vi "UI V7.1.2b.vi"() -> ()   [LabVIEW 2017]
uses:
  <vilib>/Instr/_visa.llb/VISA Configure Serial Port (Instr).vi
  <vilib>/addons/Biomedical/Biosignal Measurements/Biosignal Preprocessing/Biosignal Rate Extractor (Waveform).vi
  <vilib>/addons/Biomedical/NI_BMTK_Measurements.lvlib
panel:
  in  "?":refnum<visa-resource-name>
  out "CH2  2":waveform(i32)(graph)
  out "CH1 2":waveform(i32)(graph)
  out "led ch1":bool
  out "led ch1 2":bool
  out "CH1 PM":dbl
  out "CH1":dbl(slide) scale=0.0..255.0
  out "CH2":dbl(slide) scale=0.0..255.0
  out "CH2 PM":dbl
  out "output 2":i32
  out "output 1":i32
  in  "Stop Button":bool
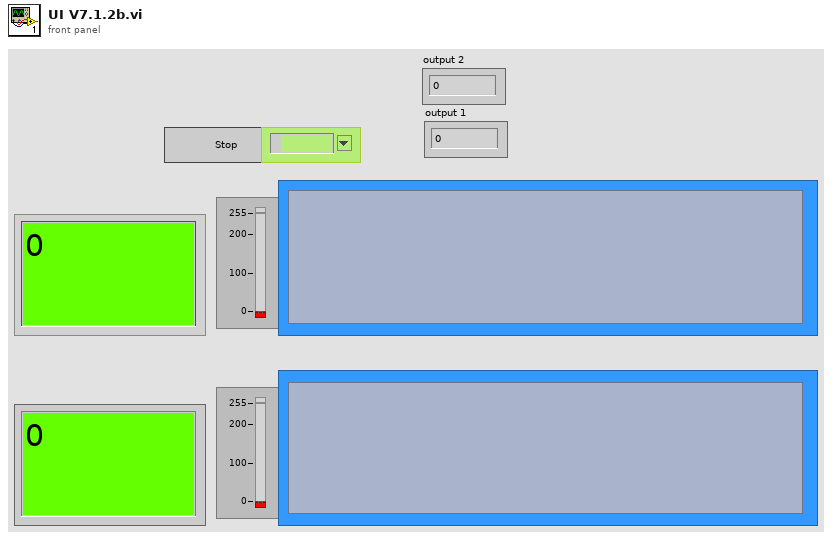
[diagram p1: front panel]
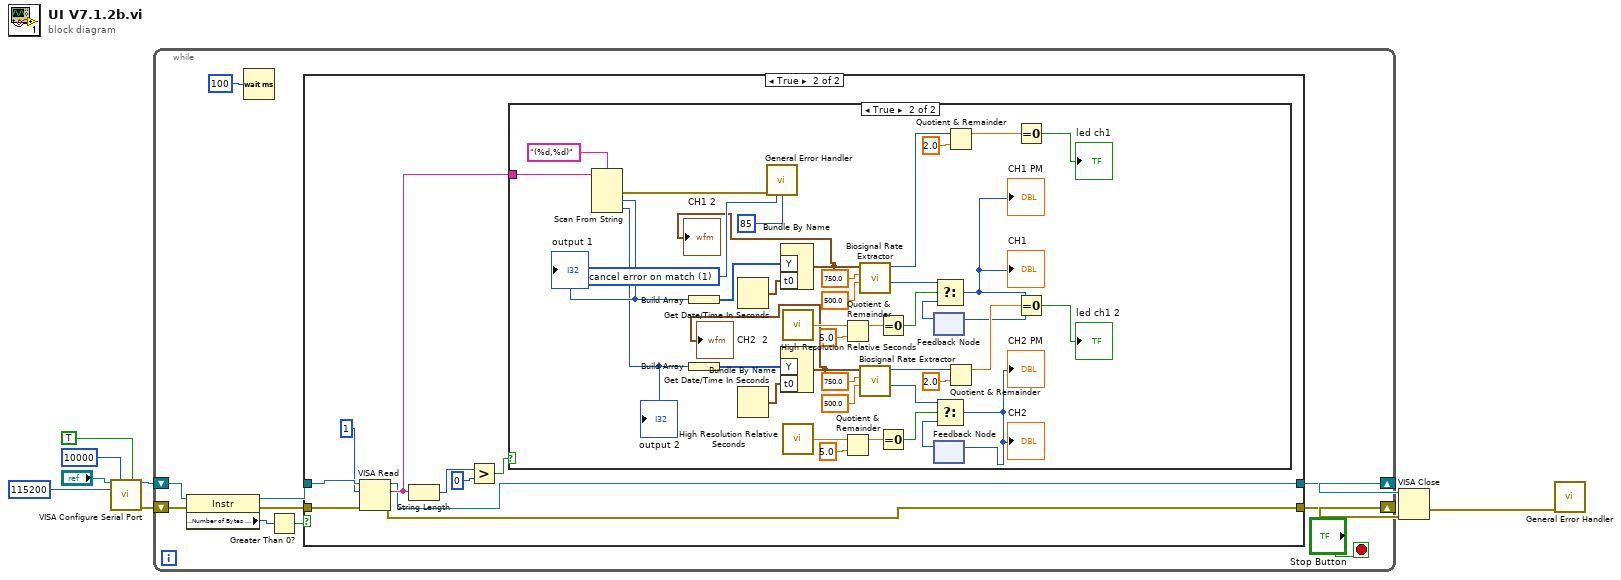
[diagram p0: block diagram]
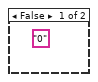
[diagram p3: hidden frame]
diagram:
  n1 = call-poly "VISA Configure Serial Port"("VISA resource name"="?", "timeout (10sec)"=u32 10000, "Enable Termination\nChar (T)"=TRUE ("Enable Termination\nChar (T)"), "baud rate (9600)"=u32 115200) -> ("VISA resource name out"=w2:refnum<visa-resource-name>, "error out"=w1:errorcluster)  [unwired: 10 in]
  n2 = while {
    shift-right: [w18] -> w7
    shift-left: w2 -> [w13]
    shift-right: [w11] -> w6
    shift-left: w1 -> [w12]
    stop <- "Stop Button" stop-if-true
    n3 = property class="Instr"(reference=w13, error in=w12) -> (reference out=w17:refnum<visa-resource-name>, error out=w16:errorcluster, "Serial Settings:Number of Bytes at Serial Port"=w15:u32)
    n4 = Wait (ms)(milliseconds to wait=u32 100) -> ()  [unwired: 1 out]
    n5 = Greater Than 0?(x=w15) -> (x > 0?=w14:bool)
    n6 = case shown="True" w14 {
      tunnel: w17 -> [w21 w30]
      tunnel: w16 -> [w20 w29]
      tunnel: [w21 w24] -> w18
      tunnel: [w20 w23] -> w11
      frame False {
      }
      frame True {
        n7 = VISA Read(VISA resource name=w30, byte count=u32 1, error in (no error)=w29) -> (VISA resource name out=w24:refnum<visa-resource-name>, read buffer=w28:string, error out=w23:errorcluster)  [unwired: 1 out]
        n8 = String Length(string=w28) -> (length=w27:i32)
        n9 = Greater?(x=w27, y=0) -> (0:w25:bool)
        n10 = case shown="True" w25 {
          tunnel: w28 -> [_ w69]
          frame False {
            (unwired) "0"
          }
          frame True {
            w67 = 1 items=["no exception", "cancel error on match", "set error on match"] ("[exception action] (none:0)")
            n11 = Scan From String(format string="(%d,%d)", input string=w69) -> (error out=w66:errorcluster, output 1=w57:i32, output 2=w35:i32)  [unwired: 4 in, 2 out]
            "output 2" <- w35
            "output 1" <- w57
            n12 = Build Array(w57) -> (w58:i32[])
            n13 = Build Array(w35) -> (w42:i32[])
            n14 = Get Date/Time In Seconds() -> (seconds since 1Jan1904=w63:timestamp)
            n15 = Get Date/Time In Seconds() -> (seconds since 1Jan1904=w37:timestamp)
            n16 = call <vilib>:"General Error Handler.vi"("error in (no error)"=w66, "[exception action] (none:0)"=w67, "[exception code]"=85) -> ()  [unwired: 8 in, 5 out]
            n17 = Bundle By Name("Y"=w58, "t0"=w63) -> (w31:waveform(i32))  [unwired: 1 in]
            "CH1 2" <- w31
            n18 = Bundle By Name("Y"=w42, "t0"=w37) -> (w32:waveform(i32))  [unwired: 1 in]
            "CH2  2" <- w32
            n19 = call <vilib>:"High Resolution Relative Seconds.vi"() -> ("relative seconds"=w53:dbl)
            n20 = call <vilib>:"High Resolution Relative Seconds.vi"() -> ("relative seconds"=w46:dbl)
            n21 = Quotient & Remainder(x=w53, y=5.0) -> (x-y*floor(x/y)=w56:dbl)  [unwired: 1 out]
            n22 = Quotient & Remainder(x=w46, y=5.0) -> (x-y*floor(x/y)=w43:dbl)  [unwired: 1 out]
            n23 = call-poly <vilib>:"Biosignal Rate Extractor.vi"("low threshold"=500.0, "high threshold"=750.0, "biosignal"=w31) -> ("number of cycles per minuets"=w54:i32, "number of cycles"=w64:i32)  [unwired: 5 in, 2 out]
            n24 = call-poly <vilib>:"Biosignal Rate Extractor.vi"("low threshold"=500.0, "high threshold"=750.0, "biosignal"=w32) -> ("number of cycles per minuets"=w45:i32, "number of cycles"=w36:i32)  [unwired: 5 in, 2 out]
            n25 = Equal To 0?(x=w56) -> (x = 0?=w55:bool)
            n26 = Equal To 0?(x=w43) -> (x = 0?=w44:bool)
            n27 = feedback #1() -> (w51:i32)  [unwired: 1 in]
            n28 = feedback #2() -> (w48:i32)  [unwired: 1 in]
            n29 = Select(t=w54, s=w55, f=w51) -> (s? t:f=w34:i32)
            "CH1 PM" <- w34
            "CH1" <- w34
            n30 = feedback-in #1(w34) -> ()
            n31 = Select(t=w45, s=w44, f=w48) -> (s? t:f=w33:i32)
            "CH2" <- w33
            "CH2 PM" <- w33
            n32 = feedback-in #2(w33) -> ()
            n33 = Quotient & Remainder(x=w64, y=2.0) -> (x-y*floor(x/y)=w62:dbl)  [unwired: 1 out]
            n34 = Quotient & Remainder(x=w36, y=2.0) -> (x-y*floor(x/y)=w38:dbl)  [unwired: 1 out]
            n35 = Equal To 0?(x=w62) -> (x = 0?=→"led ch1":bool)
            n36 = Equal To 0?(x=w38) -> (x = 0?=→"led ch1 2":bool)
          }
        }
      }
    }
  }
  n37 = VISA Close(VISA resource name=w7, error in (no error)=w6) -> (error out=w5:errorcluster)
  n38 = call <vilib>:"General Error Handler.vi"("error in (no error)"=w5) -> ()  [unwired: 10 in, 5 out]
